vi "test_scd_HVBiasVoltage.vi"(8 "error in":errorcluster, 11 "SCD in":refnum<class "SCD.lvclass">) -> (0 "error out":errorcluster, 3 "SCD out":refnum<class "SCD.lvclass">)   [LabVIEW 2023, in "horiba.test.lvlib"]
uses:
  horiba.test.lvlib
  Classes/SCD/SCD.lvclass
  C:/Projects/Horiba/horiba-labview-sdk/Source/Classes/GenericDevice/GenericDevice.lvclass
  <vilib>/addons/_JKI Toolkits/Caraya/classes/Assert/Assert Equal Value_Variant.vi
  <vilib>/addons/_JKI Toolkits/Caraya/classes/Test/Test.lvclass
  <vilib>/addons/_JKI Toolkits/Caraya/classes/Assert/Assert.lvclass
  <userlib>/_OpenG.lib/lvdata/lvdata.llb/openg_variant.lvlib
panel:
  # "Connector Pane"
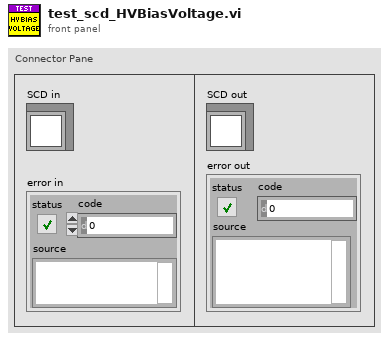
[diagram p1: front panel]
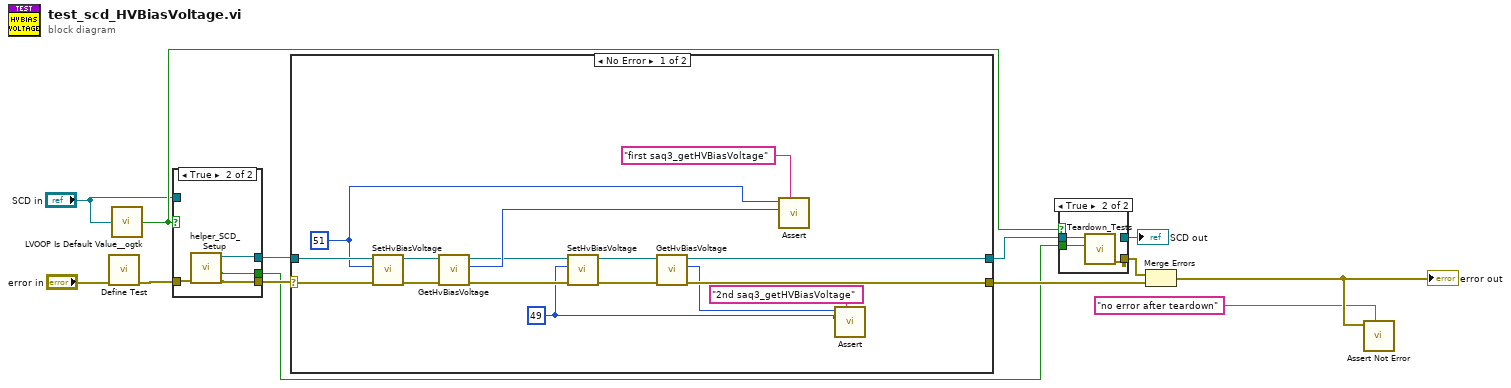
[diagram p0: block diagram]
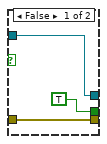
[diagram p3: hidden frame]
diagram:
  n1 = call <vilib>:"Define Test.vi"("error in (no error)"="error in") -> ("error out"=w9:errorcluster)  [unwired: 9 in, 1 out]
  n2 = call <userlib>:"LVOOP Is Default Value__ogtk.vi"("Object"="SCD in") -> ("Is Default Value?"=w3:bool)
  n3 = case shown="True" w3 {
    tunnel: w9 -> [w16 w18]
    tunnel: [w16 w20] -> w8
    tunnel: [w14 w17] -> w7
    tunnel: [TRUE ("Module Was Already Running?") w19] -> w4
    tunnel: "SCD in" -> [w14 _]
    frame False {
    }
    frame True {
      n4 = call "helper_SCD_Setup.vi"("error in"=w18) -> ("error out"=w20:errorcluster, "Module Was Already Running?"=w19:bool, "SCD out"=w17:refnum<class "SCD.lvclass">)  [unwired: 7 in, 1 out]
    }
  }
  n5 = case shown="No Error" w8 {
    selector: w8 -> [w35 w38]
    tunnel: [w24 w37] -> w12
    tunnel: w7 -> [w36 w37]
    tunnel: [w26 w38] -> w11
    frame No Error {
      w21 = 49 ("integration_time")
      w30 = 51 ("integration_time")
      n6 = call "SetHvBiasVoltage.vi"("error in (no error)"=w35, "HVBiasVoltage"=w30, "SCD in"=w36) -> ("error out"=w33:errorcluster, "SCD out"=w31:refnum<class "SCD.lvclass">)  [unwired: 7 in]
      n7 = call "GetHvBiasVoltage.vi"("error in (no error)"=w33, "SCD in"=w31) -> ("error out"=w32:errorcluster, "HVBiasVoltage"=w29:i32, "SCD out"=w27:refnum<class "SCD.lvclass">)  [unwired: 7 in]
      n8 = call "SetHvBiasVoltage.vi"("error in (no error)"=w32, "HVBiasVoltage"=w21, "SCD in"=w27) -> ("error out"=w28:errorcluster, "SCD out"=w25:refnum<class "SCD.lvclass">)  [unwired: 7 in]
      n9 = call "GetHvBiasVoltage.vi"("error in (no error)"=w28, "SCD in"=w25) -> ("error out"=w26:errorcluster, "HVBiasVoltage"=w22:i32, "SCD out"=w24:refnum<class "SCD.lvclass">)  [unwired: 7 in]
      n10 = call-poly <vilib>:"Assert.vi"("Label"="first saq3_getHVBiasVoltage", "Y"=w29, "X"=w30) -> ()  [unwired: 7 in, 2 out]
      n11 = call-poly <vilib>:"Assert.vi"("Label"="2nd saq3_getHVBiasVoltage", "Y"=w21, "X"=w22) -> ()  [unwired: 7 in, 2 out]
    }
    frame Error {
    }
  }
  n12 = case shown="True" w3 {
    tunnel: w12 -> [w39 w42]
    tunnel: [_ w41] -> w6
    tunnel: w4 -> [_ w40]
    tunnel: [w39 _] -> w1
    frame False {
    }
    frame True {
      n13 = call "Teardown_Tests.vi"("Module Was Already Running?"=w40, "horiba.lvlib:GenericDevice"=w42) -> ("error out"=w41:errorcluster)  [unwired: 8 in, 1 out]
    }
  }
  "SCD out" <- w1
  n14 = Merge Errors(w6, w11) -> (w10:errorcluster)
  "error out" <- w10
  n15 = call <vilib>:"Assert Not Error.vi"("Label"="no error after teardown", "Not Error?"=w10) -> ()  [unwired: 8 in, 2 out]
